vi "Get Device ID Config.vi"() -> (0 "error out":errorcluster, 2 "device id":i32)   [LabVIEW 2020, in "Topas.lvlib"]
uses:
  Topas.lvlib
  <vilib>/Utility/config.llb/Read Key (I32).vi
  <vilib>/Utility/config.llb/NI_LVConfig.lvlib
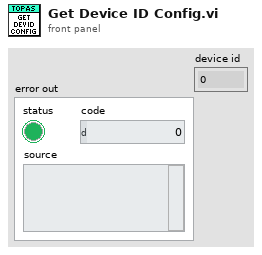
[diagram p1: front panel]
types:
  T1 = typedef "NI_LVConfig.lvlib/Config Data RefNum.ctl" = refnum<k1>
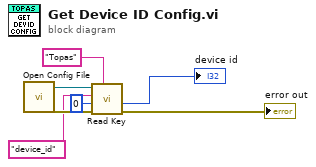
[diagram p0: block diagram]
diagram:
  n1 = call "Open Config File.vi"() -> ("error out"=w5:errorcluster, "Refnum out"=w6:T1)  [unwired: 10 in]
  n2 = call-poly <vilib>:"Read Key.vi"("section"="Topas", "error in (no error)"=w5, "default value"=0, "key"="device_id", "refnum"=w6) -> ("error out"=→"error out":errorcluster, "value"=→"device id":i32)  [unwired: 3 in, 2 out]
